vi "Extract Data from N-Channel Array (2D DBL).vi"() -> ()   [LabVIEW 2019]
uses:
  <vilib>/DAQmx/read.llb/DAQmx Read (Analog 2D DBL NChan NSamp).vi
  <vilib>/DAQmx/create/channels.llb/DAQmx Create Channel (AI-Voltage-Basic).vi
  <vilib>/DAQmx/configure/timing.llb/DAQmx Timing (Sample Clock).vi
  <vilib>/DAQmx/miscellaneous.llb/DAQmx Fill In Error Info.vi
  <resource>/objmgr/daqmx.rc
panel:
  out "Actual Sample Rate (Hz)":dbl
  in  "Desired Sample Rate (Hz)":dbl=2560.0
  in  "Number of Samples":i32=256
  in  "Stop":bool
  out "All Channels":dbl[][](graph)
  out "Indexed Channel":dbl[](graph)
  out "Subset of Channels":dbl[][](graph)
  in  "Physical Channels":tag="PCI-6221/ai0, PCI-6221/ai2:3"
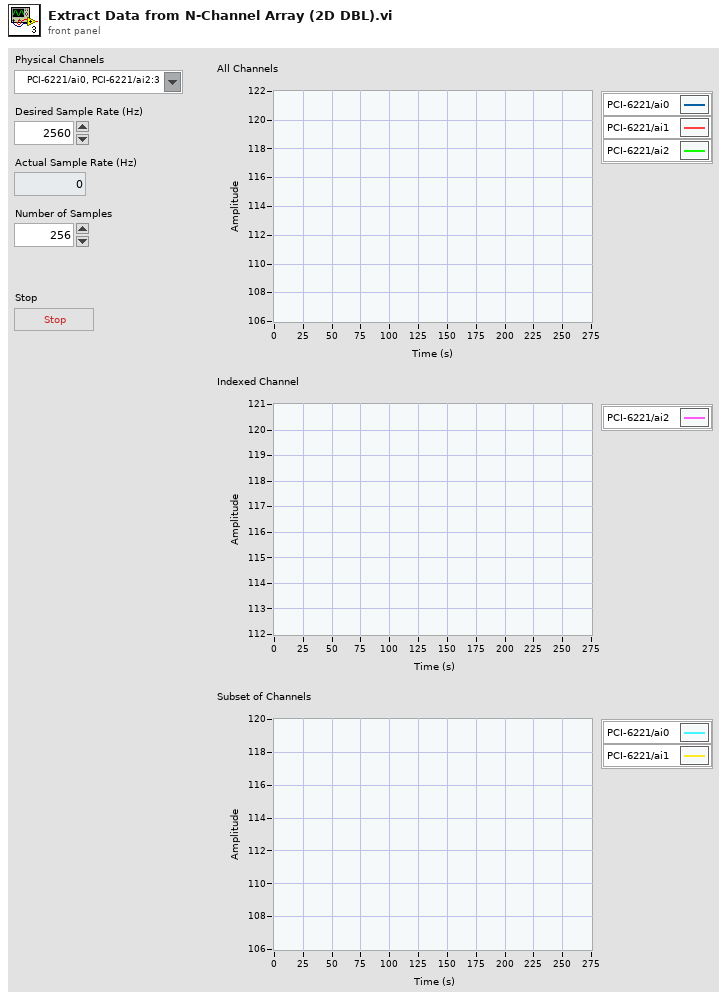
[diagram p1: front panel]
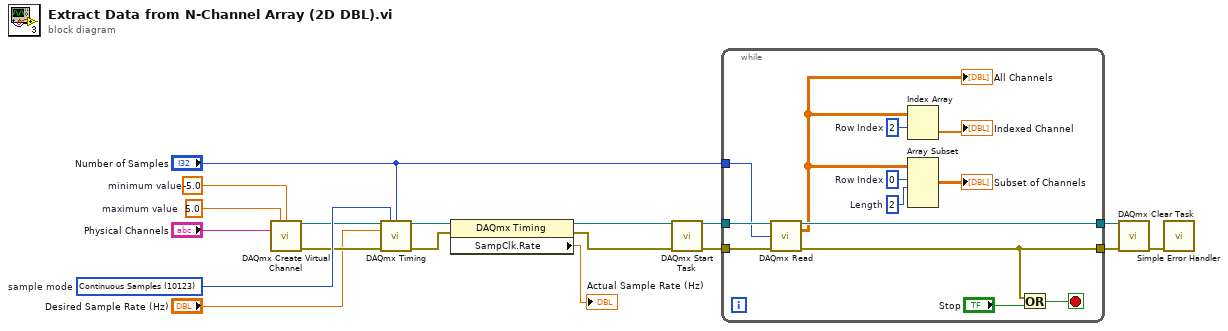
[diagram p0: block diagram]
diagram:
  w13 = 5.0  # maximum value
  w14 = -5.0  # minimum value
  w18 = 10123 items=["Finite Samples"=10178, "Continuous Samples"=10123, "Hardware Timed Single Point"=12522]  # sample mode
  n1 = call-poly <vilib>:"DAQmx Create Virtual Channel.vi"("maximum value"=w13, "minimum value"=w14, "physical channels"="Physical Channels") -> ("task out"=w17:refnum<k21>, "error out"=w16:errorcluster)  [unwired: 11 in]
  n2 = call-poly <vilib>:"DAQmx Timing.vi"("task/channels in"=w17, "sample mode"=w18, "samples per channel"="Number of Samples", "rate"="Desired Sample Rate (Hz)", "error in"=w16) -> ("task out"=w5:refnum<k21>, "error out"=w4:errorcluster)  [unwired: 9 in]
  n3 = property class="DAQmx Timing"(reference=w5, error in=w4) -> (reference out=w3:refnum<k21>, error out=w2:errorcluster, "SampClk.Rate"=→"Actual Sample Rate (Hz)":dbl)
  n4 = call <vilib>:"DAQmx Start Task.vi"("task/channels in"=w3, "error in"=w2) -> ("task out"=w9:refnum<k21>, "error out"=w8:errorcluster)  [unwired: 12 in]
  n5 = while {
    tunnel: [w31] -> w12
    tunnel: [w30] -> w11
    tunnel: w9 -> [w27]
    tunnel: w8 -> [w26]
    tunnel: "Number of Samples" -> [w25]
    stop <- w28 stop-if-true
    w20 = 2  # Length
    w21 = 0  # Row Index
    w23 = 2  # Row Index
    n6 = call-poly <vilib>:"DAQmx Read.vi"("task/channels in"=w27, "number of samples per channel"=w25, "error in"=w26) -> ("task out"=w31:refnum<k21>, "data"=w22:dbl[][], "error out"=w30:errorcluster)  [unwired: 10 in]
    "All Channels" <- w22
    n7 = Index Array "Index Array"(array=w22, index (row)=w23) -> (element=→"Indexed Channel":dbl[])  [unwired: 1 in]
    n8 = Array Subset "Array Subset"(array=w22, index (row)=w21, length (row)=w20) -> (→"Subset of Channels":dbl[][])  [unwired: 2 in]
    n9 = Or(x=w30, y="Stop") -> (x .or. y?=w28:bool)
  }
  n10 = call <vilib>:"DAQmx Clear Task.vi"("task in"=w12, "error in"=w11) -> ("error out"=w10:errorcluster)  [unwired: 13 in]
  n11 = call <vilib>:"Simple Error Handler.vi"("error in (no error)"=w10) -> ()  [unwired: 4 in, 5 out]
